vi "Read Type.vi"(8 "error in (no error)":errorcluster, 11 "Library in":refnum<class "Library.lvclass">) -> (0 "error out":errorcluster, 2 "Module type":T1, 3 "Library out":refnum<class "Library.lvclass">)   [LabVIEW 2019, in "Library.lvclass"]
uses:
  Library.lvclass
  Panther Dashboard/Module type--enum.ctl
  Panther Dashboard/Panther Dashboard.lvlib
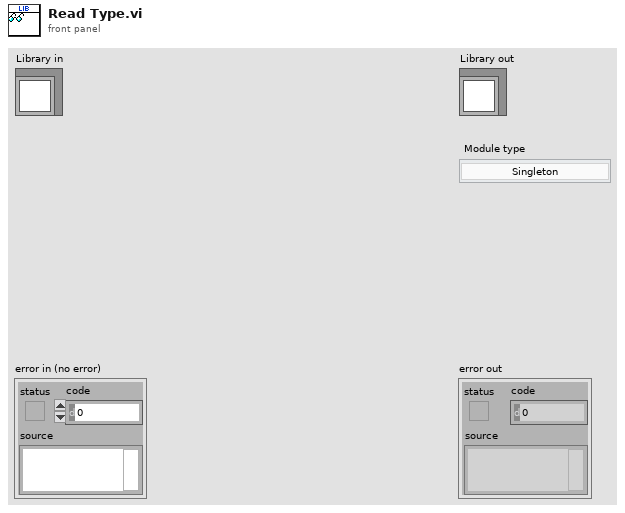
[diagram p1: front panel]
types:
  T1 = typedef "Panther Dashboard.lvlib/Module type--enum.ctl" = enum16{"Singleton", "Cloneable"}
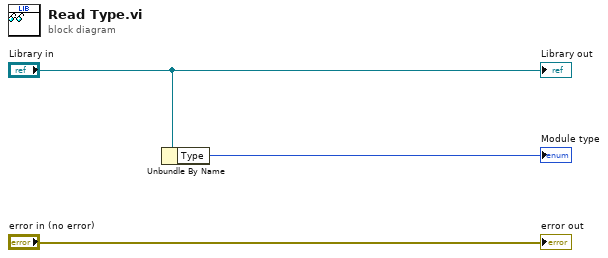
[diagram p0: block diagram]
diagram:
  n1 = Unbundle By Name("Library in") -> ("Type"=→"Module type":T1)
  "error out" <- "error in (no error)"
  "Library out" <- "Library in"
